vi "Record Results, Double Array.vi"(6 "n rows":i32=10, 7 "step name":string="Charging Results", 8 "error in":errorcluster, 9 "test case":T1, 10 "Numeric Results":dbl[](array[numeric]) format="%.2f", 11 "Sequence Context":refnum<k7>) -> (0 "error out":errorcluster, 3 "Sequence Context dup":refnum<k7>)   [LabVIEW 2010]
doc: "This function records an array of double results in the LabVIEW Master log and in TestStand.\n\nIt transfers a single Compare Data Test (CDT) record to the current TestStand sequence step."
uses:
  Active Output Test Cases.ctl
panel:
  in  "Acceptance Criteria":string[][](table) caption="Table 1"
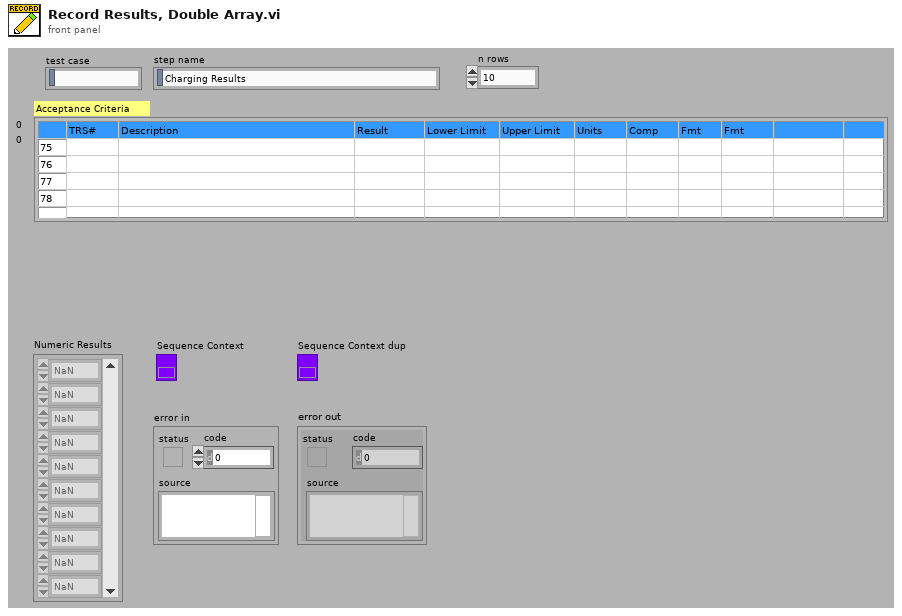
[diagram p1: front panel]
types:
  T1 = typedef "Active Output Test Cases.ctl" = string
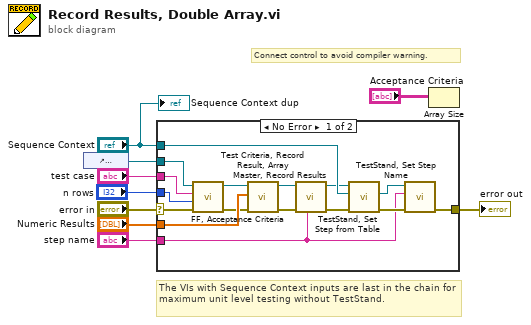
[diagram p0: block diagram]
diagram:
  # "The VIs with Sequence Context inputs are last in the chain for maximum unit level testing without TestStand."
  # "Connect control to avoid compiler warning."
  n1 = control-ref of="Acceptance Criteria"() -> (w4:refnum<vi>)
  n2 = case shown="No Error" "error in" {
    selector: "error in" -> [w23 w26]
    tunnel: [w21 w26] -> w9
    tunnel: "Sequence Context" -> [w20 _]
    tunnel: "test case" -> [w18 _]
    tunnel: w4 -> [w24 _]
    tunnel: "step name" -> [w10 _]
    tunnel: "n rows" -> [w17 _]
    tunnel: "Numeric Results" -> [w16 _]
    frame No Error {
      n3 = call "FF, Acceptance Criteria.vi"("error in"=w23, "n rows"=w17, "test case"=w18, "Tbl Refnum"=w24) -> ("error out"=w15:errorcluster, "Tbl Refnum out"=w25:refnum<vi>)  [unwired: 6 in]
      n4 = call "Test Criteria, Record Result, Array.vi"("error in"=w15, "Results"=w16, "Tbl Refnum"=w25) -> ("error out"=w13:errorcluster, "Tbl Refnum out"=w14:refnum<vi>)  [unwired: 6 in, 1 out]
      n5 = call "Master, Record Results.vi"("step name"=w10, "error in"=w13, "Tbl Refnum"=w14) -> ("error out"=w12:errorcluster, "Tbl Refnum dup"=w11:refnum<vi>)  [unwired: 7 in]
      n6 = call "TestStand, Set Step from Table.vi"("error in"=w12, "Sequence Context"=w20, "Tbl Refnum"=w11) -> ("error out"=w22:errorcluster, "Sequence Context Out"=w19:refnum<k7>)  [unwired: 6 in, 1 out]
      n7 = call "TestStand, Set Step Name.vi"("error in"=w22, "Step Name"=w10, "Sequence Context"=w19) -> ("error out"=w21:errorcluster)  [unwired: 7 in, 1 out]
    }
    frame Error {
    }
  }
  "error out" <- w9
  n8 = Array Size(array="Acceptance Criteria") -> ()  [unwired: 1 out]
  "Sequence Context dup" <- "Sequence Context"
